vi "get slow timing.vi"(8 "error in (no error)":errorcluster, 11 "ImagingModeSPIM in":refnum<class "ImagingModeSPIM.lvclass">) -> (0 "error out":errorcluster, 1 "frame rate":i32, 2 "dt times sampels":i32, 3 "ImagingModeSPIM out":refnum<class "ImagingModeSPIM.lvclass">)   [LabVIEW 2012, in "ImagingModeSPIM.lvclass"]
uses:
  ImagingModeSPIM.lvclass
  ImagingModeSPIM.lvclass/ImagingModeSPIM.ctl
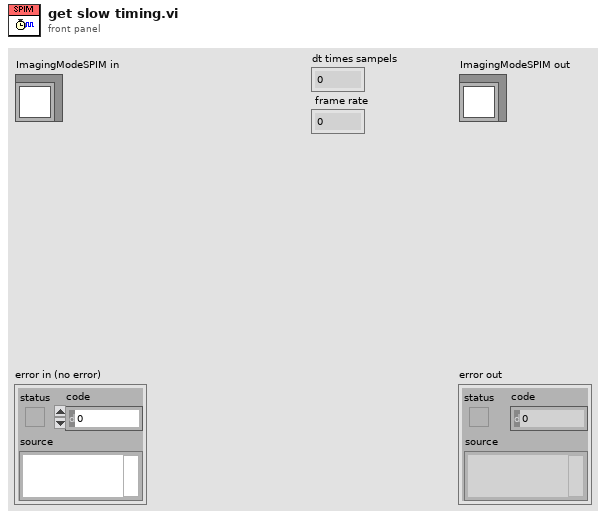
[diagram p1: front panel]
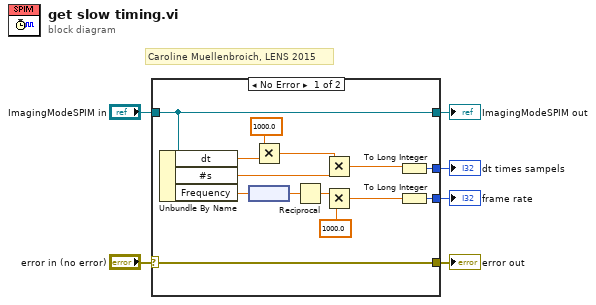
[diagram p0: block diagram]
diagram:
  # "Caroline Muellenbroich, LENS 2015"
  n1 = case shown="No Error" "error in (no error)" {
    selector: "error in (no error)" -> [w20 w22]
    tunnel: [w20 w22] -> w5
    tunnel: [w19 w21] -> w3
    tunnel: "ImagingModeSPIM in" -> [w19 w21]
    tunnel: [w16 _] -> w2
    tunnel: [w10 _] -> w1
    frame No Error {
      n2 = Unbundle By Name(w19) -> ("dt"=w9:dbl, "#s"=w18:dbl, "Frequency"=w11:dbl[unit])
      n3 = node(w11) -> (w13:dbl)
      n4 = Multiply(x=1000.0, y=w9) -> (x*y=w7:dbl)
      n5 = Reciprocal(x=w13) -> (1/x=w15:dbl)
      n6 = Multiply(x=w7, y=w18) -> (x*y=w17:dbl)
      n7 = Multiply(x=w15, y=1000.0) -> (x*y=w12:dbl)
      n8 = To Long Integer(number=w17) -> (32bit integer=w16:i32)
      n9 = To Long Integer(number=w12) -> (32bit integer=w10:i32)
    }
    frame Error {
    }
  }
  "error out" <- w5
  "ImagingModeSPIM out" <- w3
  "dt times sampels" <- w2
  "frame rate" <- w1
